vi "Parse Recursive.vi"(7 "Variant":variant, 8 "error in (no error)":errorcluster, 9 "Level":u32, 11 "String":string) -> (0 "error out":errorcluster, 3 "Remaining String":string, 5 "Variant out":variant)   [LabVIEW 2015, in "YAML Parser.lvclass"]
uses:
  YAML Parser.lvclass
  YAML Internal Type.ctl
  <vilib>/Utility/error.llb/Error Cluster From Error Code.vi
  <vilib>/ErrorRing/Error Ring.xnode
panel:
  out "String en Cours d'Analyse":string
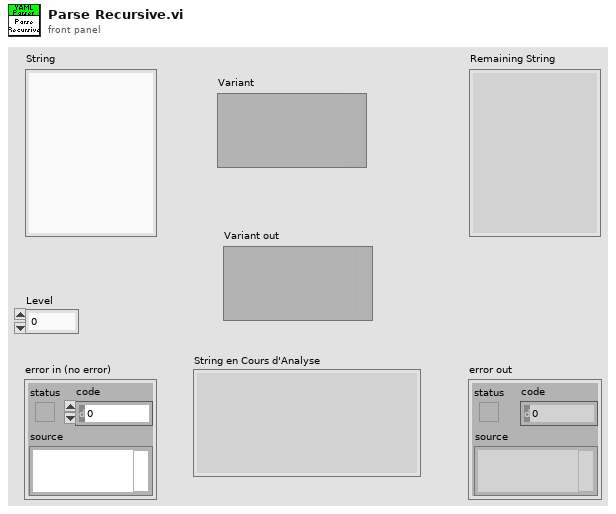
[diagram p1: front panel]
types:
  T1 = typedef "YAML Parser.lvclass/YAML Internal Type.ctl" = enum16{"Comment", "Null", "Value", "Multilines Value", "Object", "Array", "Reference", "Array Element", "Empty Line", "Key"}
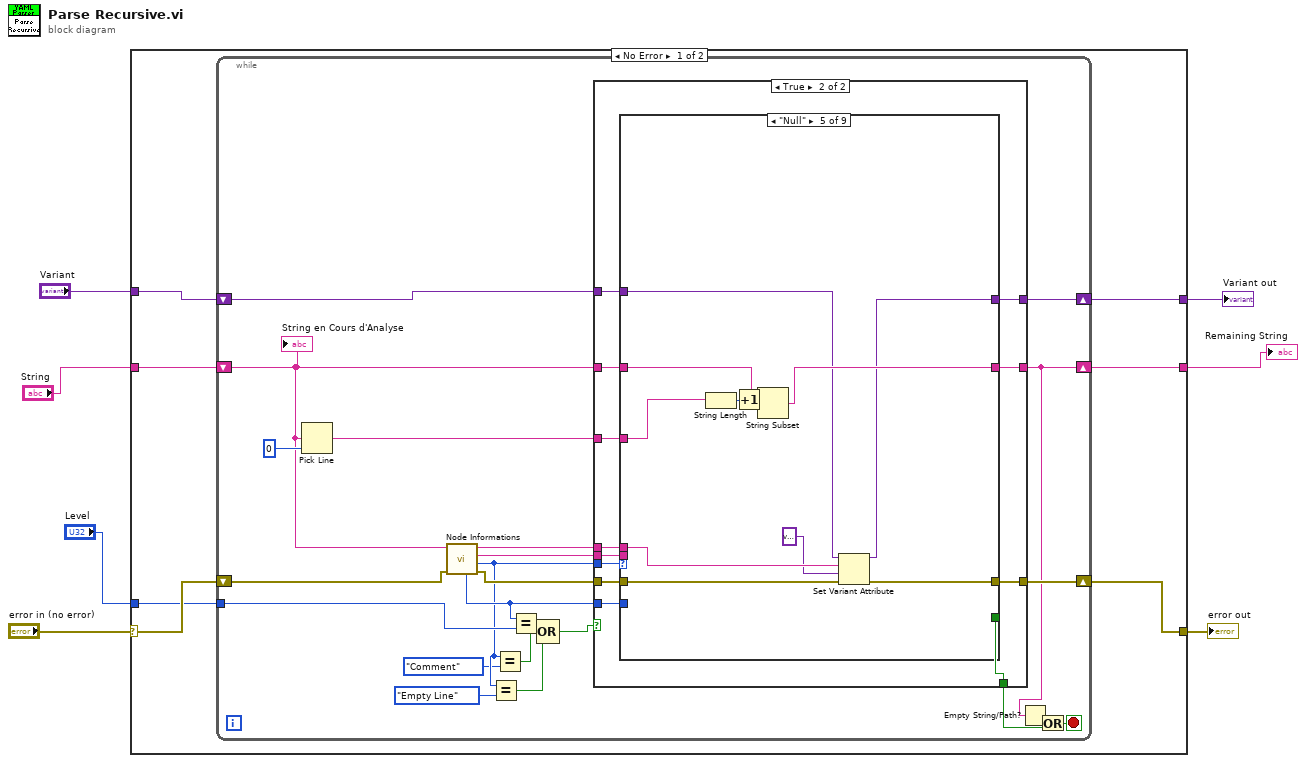
[diagram p0: block diagram]
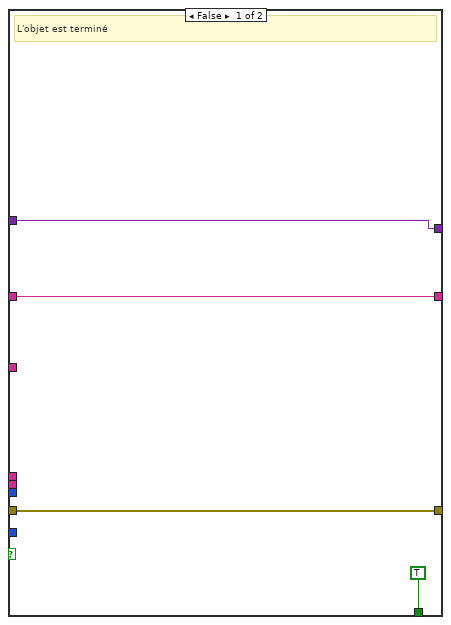
[diagram p2: hidden frame]
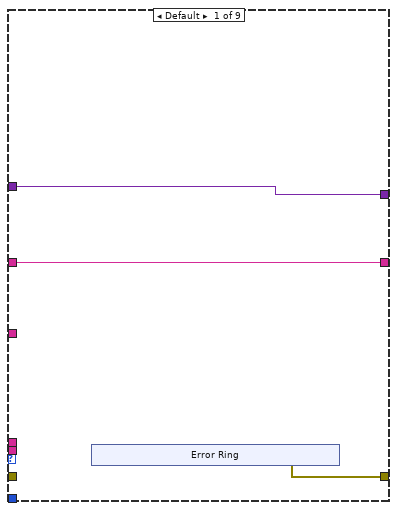
[diagram p3: hidden frame]
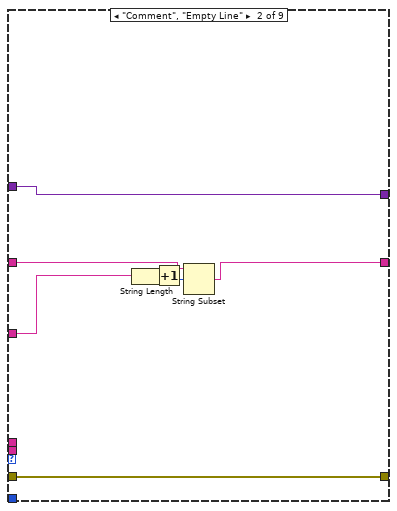
[diagram p4: hidden frame]
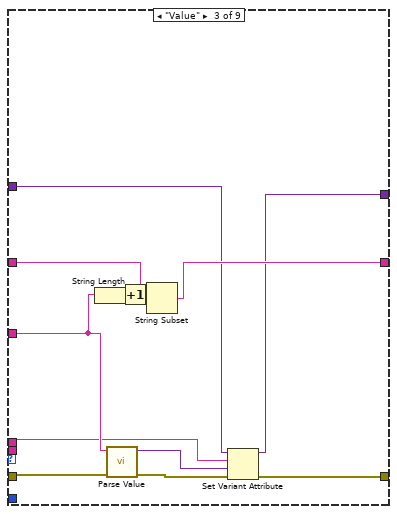
[diagram p5: hidden frame]
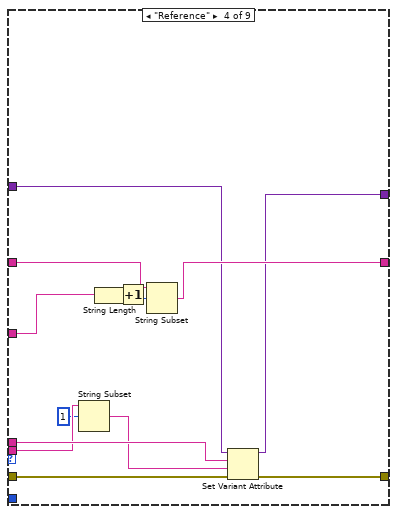
[diagram p6: hidden frame]
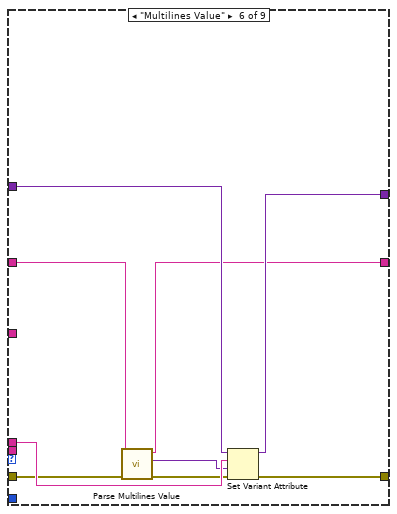
[diagram p7: hidden frame]
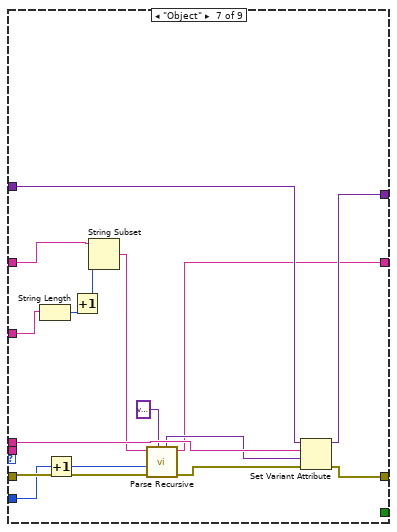
[diagram p8: hidden frame]
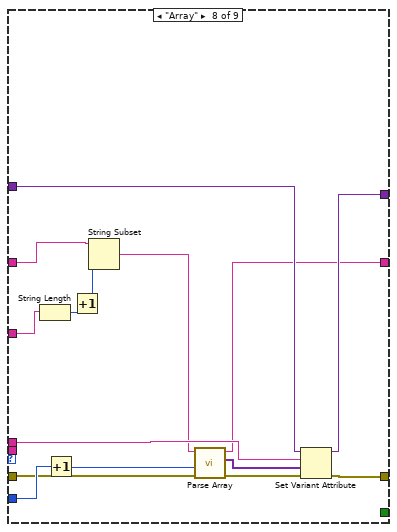
[diagram p9: hidden frame]
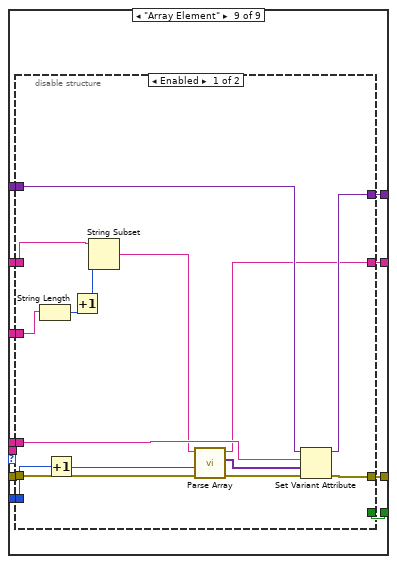
[diagram p10: hidden frame]
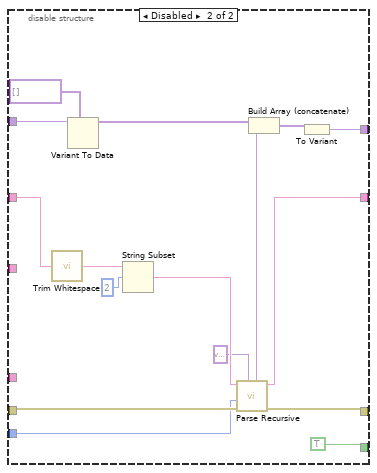
[diagram p11: hidden frame]
diagram:
  n1 = case shown="No Error" "error in (no error)" {
    selector: "error in (no error)" -> [w14 w188]
    tunnel: [w13 w188] -> w6
    tunnel: [w11 w187] -> w4
    tunnel: "String" -> [w12 w187]
    tunnel: "Variant" -> [w10 w186]
    tunnel: [w9 w186] -> w2
    tunnel: "Level" -> [w8 _]
    frame No Error {
      n2 = while {
        tunnel: w8 -> [w27]
        shift-right: [w34] -> w13
        shift-left: w14 -> [w36]
        shift-right: [w24] -> w11
        shift-left: w12 -> [w21]
        shift-right: [w30] -> w9
        shift-left: w10 -> [w31]
        stop <- w23 stop-if-true
        n3 = Pick Line(multi-line string=w21, line index=0) -> (output string=w32:string)  [unwired: 1 in]
        n4 = call "Node Informations.vi"("error in (no error)"=w36, "String"=w21) -> ("error out"=w35:errorcluster, "YAML Internal Type"=w17:T1, "Value"=w29:string, "Key"=w33:string, "Level"=w28:u32)  [unwired: 5 in]
        n5 = Equal?(x=w17, y=YAML_Internal_Type."Empty Line") -> (x = y?=w18:bool)
        n6 = Equal?(x=w17, y=YAML_Internal_Type."Comment") -> (x = y?=w19:bool)
        n7 = Equal?(x=w28, y=w27) -> (x = y?=w26:bool)
        n8 = Compound Arithmetic op=OR(w26, w19, w18) -> (w20:bool)
        n9 = case shown="True" w20 {
          tunnel: w35 -> [w39 w53]
          tunnel: [w39 w52] -> w34
          tunnel: w33 -> [_ w51]
          tunnel: w32 -> [_ w50]
          tunnel: w21 -> [w40 w49]
          tunnel: [w40 w48] -> w24
          tunnel: w31 -> [w41 w47]
          tunnel: [w41 w46] -> w30
          tunnel: w17 -> [_ w45]
          tunnel: w29 -> [_ w44]
          tunnel: w28 -> [_ w43]
          tunnel: [TRUE w42] -> w22
          frame False {
            # "L'objet est terminé"
          }
          frame True {
            n10 = case shown="\"Null\"" w45 {
              tunnel: w53 -> [_ w64 w80 w93 w104 w108 w126 w135 w147]
              tunnel: [w54 w64 w74 w88 w99 w113 w127 w142 w152] -> w52
              tunnel: w51 -> [_ _ w71 w85 w96 w110 w124 w141 w151]
              tunnel: w50 -> [_ w62 w76 w89 w100 _ w116 w137 w148]
              tunnel: w49 -> [w55 w65 w79 w92 w103 w105 w117 w138 w149]
              tunnel: [w55 w66 w77 w90 w101 w109 w121 w131 w146] -> w48
              tunnel: w47 -> [w56 w68 w73 w87 w98 w112 w129 w144 w154]
              tunnel: [w56 w68 w72 w86 w97 w111 w128 w143 w153] -> w46
              tunnel: w44 -> [_ _ _ w84 _ _ _ _ _]
              tunnel: w43 -> [_ _ _ _ _ _ w120 w140 w150]
              tunnel: [_ _ _ _ _ _ _ _ w145] -> w42
              frame Default {
                n11 = xnode "Error Ring"() -> ("error out"=w54:errorcluster)
              }
              frame "Comment", "Empty Line" {
                n12 = String Length(string=w62) -> (length=w67:i32)
                n13 = Increment(x=w67) -> (x+1=w63:i32)
                n14 = String Subset(string=w65, offset (0)=w63) -> (substring=w66:string)  [unwired: 1 in]
              }
              frame "Value" {
                n15 = String Length(string=w76) -> (length=w78:i32)
                n16 = call "Parse Value.vi"("error in (no error)"=w80, "String"=w76) -> ("error out"=w75:errorcluster, "Value"=w70:variant)  [unwired: 8 in]
                n17 = Increment(x=w78) -> (x+1=w69:i32)
                n18 = String Subset(string=w79, offset (0)=w69) -> (substring=w77:string)  [unwired: 1 in]
                n19 = Set Variant Attribute(Variant=w73, name=w71, value=w70, error in=w75) -> (Variant out=w72:variant, error out=w74:errorcluster)  [unwired: 1 out]
              }
              frame "Reference" {
                n20 = String Subset(string=w84, offset (0)=1) -> (substring=w82:string)  [unwired: 1 in]
                n21 = String Length(string=w89) -> (length=w91:i32)
                n22 = Increment(x=w91) -> (x+1=w81:i32)
                n23 = String Subset(string=w92, offset (0)=w81) -> (substring=w90:string)  [unwired: 1 in]
                n24 = Set Variant Attribute(Variant=w87, name=w85, value=w82, error in=w93) -> (Variant out=w86:variant, error out=w88:errorcluster)  [unwired: 1 out]
              }
              frame "Null" {
                n25 = String Length(string=w100) -> (length=w102:i32)
                n26 = Increment(x=w102) -> (x+1=w95:i32)
                n27 = String Subset(string=w103, offset (0)=w95) -> (substring=w101:string)  [unwired: 1 in]
                n28 = Set Variant Attribute(Variant=w98, name=w96, value=variant, error in=w104) -> (Variant out=w97:variant, error out=w99:errorcluster)  [unwired: 1 out]
              }
              frame "Multilines Value" {
                n29 = call "Parse Multilines Value.vi"("error in (no error)"=w108, "String"=w105) -> ("error out"=w107:errorcluster, "Value"=w106:variant, "Remaining String"=w109:string)  [unwired: 7 in]
                n30 = Set Variant Attribute(Variant=w112, name=w110, value=w106, error in=w107) -> (Variant out=w111:variant, error out=w113:errorcluster)  [unwired: 1 out]
              }
              frame "Object" {
                n31 = String Length(string=w116) -> (length=w118:i32)
                n32 = Increment(x=w120) -> (x+1=w119:u32)
                n33 = Increment(x=w118) -> (x+1=w114:i32)
                n34 = String Subset(string=w117, offset (0)=w114) -> (substring=w115:string)  [unwired: 1 in]
                n35 = call "Parse Recursive.vi"("Variant"=variant, "error in (no error)"=w126, "Level"=w119, "String"=w115) -> ("error out"=w125:errorcluster, "Remaining String"=w121:string, "Variant out"=w123:variant)  [unwired: 5 in]
                n36 = Set Variant Attribute(Variant=w129, name=w124, value=w123, error in=w125) -> (Variant out=w128:variant, error out=w127:errorcluster)  [unwired: 1 out]
              }
              frame "Array" {
                n37 = String Length(string=w137) -> (length=w139:i32)
                n38 = Increment(x=w140) -> (x+1=w130:u32)
                n39 = Increment(x=w139) -> (x+1=w136:i32)
                n40 = String Subset(string=w138, offset (0)=w136) -> (substring=w132:string)  [unwired: 1 in]
                n41 = call "Parse Array.vi"("error in (no error)"=w135, "Level"=w130, "String"=w132) -> ("error out"=w134:errorcluster, "Value"=w133:variant[], "Remaining String"=w131:string)  [unwired: 6 in]
                n42 = Set Variant Attribute(Variant=w144, name=w141, value=w133, error in=w134) -> (Variant out=w143:variant, error out=w142:errorcluster)  [unwired: 1 out]
              }
              frame "Array Element" {
                n43 = disable-structure shown="Enabled" {
                  disable-tunnel: w154 -> [w169 w176]
                  disable-tunnel: [w168 w171] -> w153
                  disable-tunnel: [w167 w177] -> w152
                  disable-tunnel: w151 -> [w166 _]
                  disable-tunnel: w150 -> [w165 w180]
                  disable-tunnel: w149 -> [w163 w183]
                  disable-tunnel: w148 -> [w162 _]
                  disable-tunnel: w147 -> [w160 w182]
                  disable-tunnel: [w156 w178] -> w146
                  disable-tunnel: [_ TRUE] -> w145
                  frame Enabled {
                    n44 = String Length(string=w162) -> (length=w164:i32)
                    n45 = Increment(x=w165) -> (x+1=w155:u32)
                    n46 = Increment(x=w164) -> (x+1=w161:i32)
                    n47 = String Subset(string=w163, offset (0)=w161) -> (substring=w157:string)  [unwired: 1 in]
                    n48 = call "Parse Array.vi"("error in (no error)"=w160, "Level"=w155, "String"=w157) -> ("error out"=w159:errorcluster, "Value"=w158:variant[], "Remaining String"=w156:string)  [unwired: 6 in]
                    n49 = Set Variant Attribute(Variant=w169, name=w166, value=w158, error in=w159) -> (Variant out=w168:variant, error out=w167:errorcluster)  [unwired: 1 out]
                  }
                  frame Disabled {
                    n50 = call <vilib>:"Trim Whitespace.vi"("string"=w183) -> ("trimmed string"=w185:string)  [unwired: 1 in]
                    n51 = Variant To Data(type=variant[] [], Variant=w176) -> (data=w174:variant[])  [unwired: 1 in, 1 out]
                    n52 = String Subset(string=w185, offset (0)=2 ("length (rest)")) -> (substring=w181:string)  [unwired: 1 in]
                    n53 = call "Parse Recursive.vi"("Variant"=variant, "error in (no error)"=w182, "Level"=w180, "String"=w181) -> ("error out"=w177:errorcluster, "Remaining String"=w178:string, "Variant out"=w173:variant)  [unwired: 5 in]
                    n54 = Build Array (concatenate)(w174, w173) -> (w172:variant[])
                    n55 = To Variant(anything=w172) -> (Variant=w171:variant)
                  }
                }
              }
            }
          }
        }
        n56 = Empty String/Path?(string/path=w24) -> (empty?=w25:bool)
        n57 = Or(x=w25, y=w22) -> (x .or. y?=w23:bool)
        "String en Cours d'Analyse" <- w21
      }
    }
    frame Error {
    }
  }
  "error out" <- w6
  "Remaining String" <- w4
  "Variant out" <- w2
